vi "diff_x3.vi"() -> ()   [LabVIEW 2014]
panel:
  in  "diff_x3":dbl
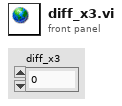
[diagram p1: front panel]
diagram:
